vi "Subpanel_GetViRefs.vi"(1 "Path":path, 2 "Command":enum16{"load", "init", "destroyAll"}(ring)=enum."init", 5 "error in (no error)":errorcluster) -> (14 "VIRef":refnum<vi>, 17 "CreatedNew":bool, 19 "error out":errorcluster)   [LabVIEW 2016]
doc: "Speicher VI welches die Subpanels erstellt und dessen Referenzen speichert\ninit: leert Speicher\nload: lädt ein Subpanel anhand Pfad\ndestroyAll: schliesst alle offenen Subpanels\n\n16.10.14 7 sige"
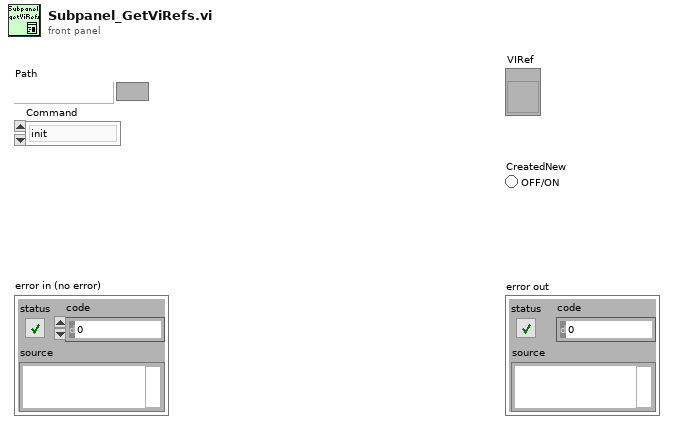
[diagram p1: front panel]
types:
  T1 = cluster{"Path":path, "vi reference":refnum<vi>}[]
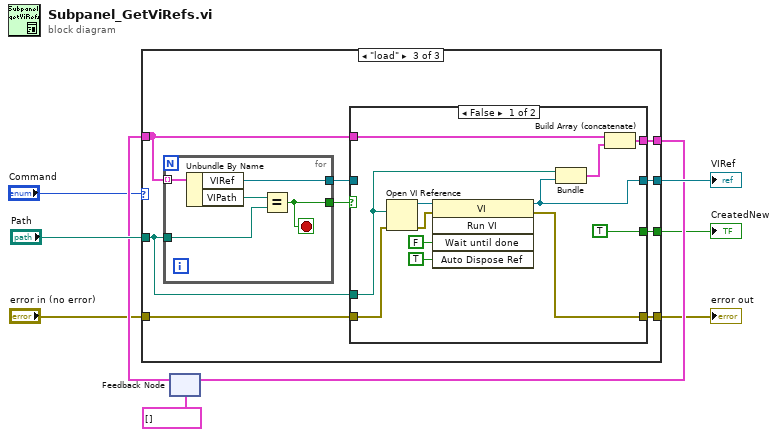
[diagram p0: block diagram]
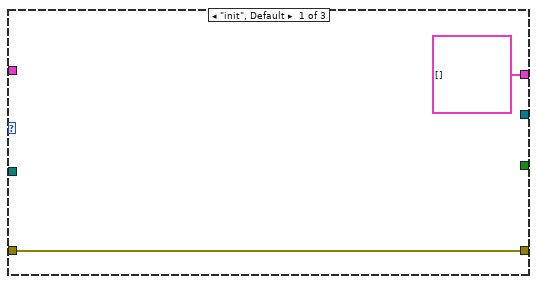
[diagram p2: hidden frame]
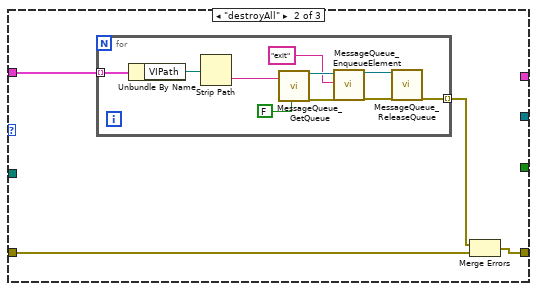
[diagram p3: hidden frame]
diagram:
  n1 = feedback #1(cluster{"VIPath":path, "VIRef":refnum<vi>}[] []) -> (w6:cluster{"VIPath":path, "VIRef":refnum<vi>}[])
  n2 = case shown="\"load\"" "Command" {
    tunnel: "Path" -> [_ _ w29]
    tunnel: [_ _ w32] -> w8
    tunnel: [cluster{"VIPath":path, "VIRef":refnum<vi>}[] [] _ w31] -> w7
    tunnel: w6 -> [_ w15 w30]
    tunnel: [_ _ w28] -> w3
    tunnel: [w10 w13 w27] -> w2
    tunnel: "error in (no error)" -> [w10 w14 w26]
    frame "init", Default {
    }
    frame "destroyAll" {
      n3 = for {
        tunnel: w15 -> [w25] mode=indexing
        tunnel: [w16] -> w12 mode=indexing
        n4 = Unbundle By Name(w25) -> ("VIPath"=w24:path)
        n5 = Strip Path(path=w24) -> (name=w21:string)  [unwired: 1 out]
        n6 = call "MessageQueue_GetQueue.vi"("Name"=w21, "CreatIfNotFount (T)"=FALSE) -> ("QueueOut"=w22:refnum<queue>, "ErrorOut"=w19:errorcluster)  [unwired: 15 in, 1 out]
        n7 = call "MessageQueue_EnqueueElement.vi"("QueueIn"=w22, "Message"="exit", "ErrorIn"=w19) -> ("QueueOut"=w23:refnum<queue>, "ErrorOut"=w18:errorcluster)  [unwired: 15 in]
        n8 = call "MessageQueue_ReleaseQueue.vi"("QueueIn"=w23, "ErrorIn"=w18) -> ("ErrorOut"=w16:errorcluster)  [unwired: 15 in, 2 out]
      }
      n9 = Merge Errors(w12, w14) -> (w13:errorcluster)
    }
    frame "load" {
      n10 = for {
        tunnel: w30 -> [w54] mode=indexing
        tunnel: w29 -> [w52]
        tunnel: [w51] -> w34
        tunnel: [w50] -> w33
        stop <- w51 stop-if-true
        n11 = Unbundle By Name(w54) -> ("VIRef"=w50:refnum<vi>, "VIPath"=w53:path)
        n12 = Equal?(x=w53, y=w52) -> (x = y?=w51:bool)
      }
      n13 = case shown="False" w34 {
        tunnel: w33 -> [_ w49]
        tunnel: [w40 w49] -> w32
        tunnel: w30 -> [w46 w47]
        tunnel: [w45 w47] -> w31
        tunnel: w29 -> [w41 _]
        tunnel: [TRUE _] -> w28
        tunnel: [w38 w48] -> w27
        tunnel: w26 -> [w37 w48]
        frame False {
          n14 = Open VI Reference(vi path=w41, error in (no error)=w37) -> (vi reference=w43:refnum<vi>, error out=w36:errorcluster)  [unwired: 4 in]
          n15 = invoke class="VI" method="Run VI"(reference=w43, error in=w36, "Wait until done"=FALSE ("Wait Until Done"), "Auto Dispose Ref"=TRUE ("Auto Dispose Reference")) -> (reference out=w40:refnum<vi>, error out=w38:errorcluster)  [unwired: 1 in, 3 out]
          n16 = Bundle("Path"=w41, "vi reference"=w40) -> (w44:cluster{"Path":path, "vi reference":refnum<vi>})  [unwired: 1 in]
          n17 = Build Array (concatenate)(w46, w44) -> (w45:T1)
        }
        frame True {
        }
      }
    }
  }
  "VIRef" <- w8
  "CreatedNew" <- w3
  "error out" <- w2
  n18 = feedback-in #1(w7) -> ()
